vi "Test - Draw Horizontal Line.vi"() -> ()   [LabVIEW 2022 SP3, in "Raster.lvlib"]
uses:
  Raster.lvlib
  Point 2D (I32).ctl
  Utility/Utility.lvlib
  Rectangle Dimensions.ctl
  <vilib>/Analysis/NI_AALBase.lvlib
  <vilib>/Analysis/baseanly.llb/Mean (DBL).vi
  c00b0a22-0810-4ff6-887a-7b90f6060769.vi
  162ecd10-8361-4378-b30a-0faa14fefb2f.vi
  Method.ctl
panel:
  out "Delta Time [s]":dbl format="%.3p"
  out "new picture":picture
  # "(0,0)"
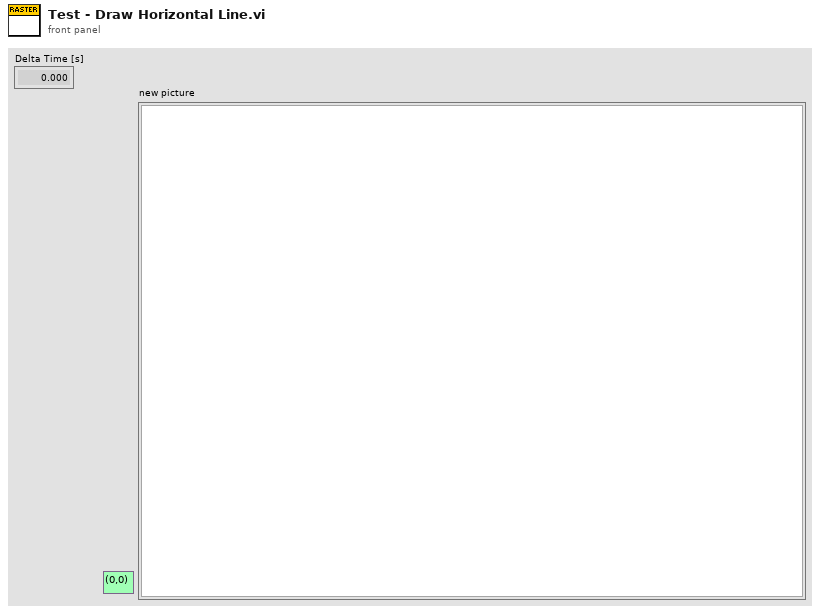
[diagram p1: front panel]
types:
  T1 = typedef "Raster.lvlib/Rectangle Dimensions.ctl" = cluster{"Width":u32, "Height":u32}
  T2 = typedef "Raster.lvlib/Point 2D (I32).ctl" = cluster{"x":i32, "y":i32}
  T3 = typedef "Raster.lvlib/Method.ctl" = enum16{"Per item", "Row", "Replace Array Subset", "MoveBlock", " MoveBlock2 "}
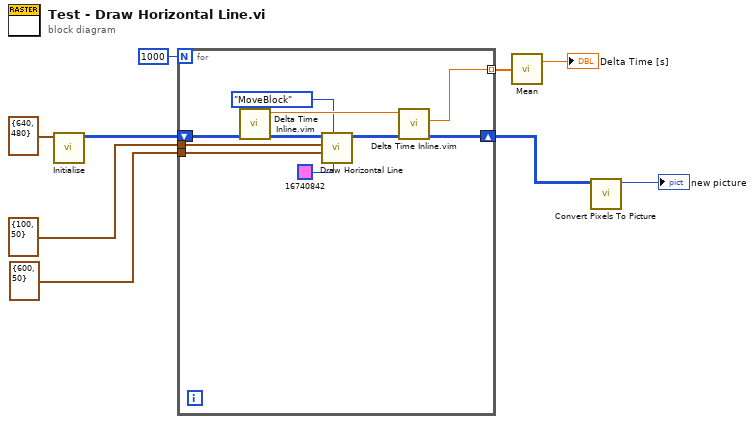
[diagram p0: block diagram]
diagram:
  n1 = call "Initialise.vi"("Screen Dimensions"=T1 {"Width"=640, "Height"=480}) -> ("Pixel Data out"=w9:u32[][])  [unwired: 10 in]
  n2 = for {
    N: 1000 -> [_]
    tunnel: T2 {"x"=100, "y"=50} ("Point 1") -> [w19]
    tunnel: T2 {"x"=600, "y"=50} ("Point 1") -> [w18]
    tunnel: [w11] -> w2 mode=indexing
    shift-right: [w13] -> w6
    shift-left: w9 -> [w16]
    n3 = call "Delta Time Inline.vim"("value in"=w16) -> ("value out"=w15:u32[][], "Relative Seconds out [s]"=w12:dbl)  [unwired: 8 in, 1 out]
    n4 = call "Draw Horizontal Line.vi"("Colour"=u32 16740842, "Method"=Method."MoveBlock", "Point 2"=w18, "Point 1"=w19, "Pixel Data in"=w15) -> ("Pixel Data out"=w14:u32[][])  [unwired: 6 in]
    n5 = call "Delta Time Inline.vim"("value in"=w14, "Relative Seconds in [s]"=w12) -> ("value out"=w13:u32[][], "Delta Time [s]"=w11:dbl)  [unwired: 7 in, 1 out]
  }
  n6 = call-poly <vilib>:"Mean.vi"("X"=w2) -> ("mean"=→"Delta Time [s]":dbl)  [unwired: 1 out]
  n7 = call "Convert Pixels To Picture.vi"("Pixel Data in"=w6) -> ("2D Picture"=→"new picture":picture)  [unwired: 9 in, 1 out]
